vi "niRFUtil LCAPI Copy WFM (1 SGL).vi"(0 "Waveform In":T1 {"y" min=0 max=127 format="%.2f"; "dx" format="%^.2e"; "x0" format="%^.2e"}, 11 "error in (no error)":errorcluster, 12 "Data Copy Descriptor":u64, 13 "Ignore Data Copy Descriptor":bool) -> (4 "Waveform Out":T1 {"y" min=0 max=127 format="%.2f"; "dx" format="%^.2e"; "x0" format="%^.2e"}, 15 "error out":errorcluster)   [LabVIEW 2015, in "niRFUtil.lvlib"]
uses:
  niRFUtil.lvlib
  Includes/niRFUtil INC Real Waveform.ctl
  Includes/niRFUtil INC Real Array.ctl
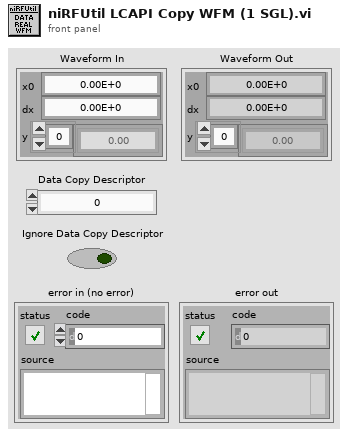
[diagram p1: front panel]
types:
  T1 = typedef "niRFUtil.lvlib/niRFUtil INC Real Waveform.ctl" = cluster{"x0":dbl, "dx":dbl, "y":T2}
  T2 = typedef "niRFUtil.lvlib/niRFUtil INC Real Array.ctl" = sgl[]
  T3 = cluster{"status":bool, "return type":i32, "errorString":string}
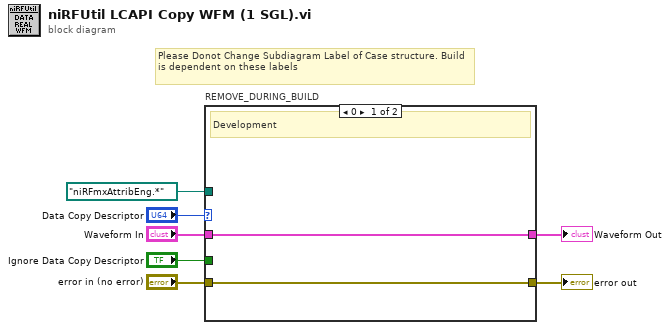
[diagram p0: block diagram]
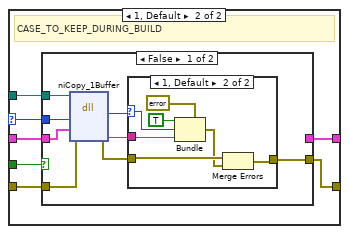
[diagram p2: hidden frame]
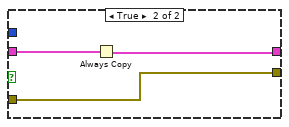
[diagram p4: hidden frame]
diagram:
  # "Please Donot Change Subdiagram Label of Case structure. Build is dependent on these labels"
  n1 = case "REMOVE_DURING_BUILD" shown="0" "Data Copy Descriptor" {
    selector: "Data Copy Descriptor" -> [_ w12]
    tunnel: "Waveform In" -> [w8 w16]
    tunnel: "error in (no error)" -> [w9 w15]
    tunnel: [w8 w14] -> w5
    tunnel: "Ignore Data Copy Descriptor" -> [_ w13]
    tunnel: [w9 w11] -> w2
    tunnel: path "niRFmxAttribEng.*" ("path in") -> [_ w10]
    frame 0 {
      # "Development"
    }
    frame 1, Default {
      # "CASE_TO_KEEP_DURING_BUILD"
      n2 = case shown="False" w13 {
        tunnel: w15 -> [w24 w35]
        tunnel: w16 -> [w23 w33]
        tunnel: w12 -> [w22 _]
        tunnel: [w18 w35] -> w11
        tunnel: [_ w34] -> w14
        tunnel: w10 -> [w17 _]
        frame False {
          n3 = dll-call lib="niRFmxAttribEng.*" fn="niCopy_1Buffer"(path in=w17, error in=w24, "dataCopyDescriptor"=w22, "source"=w23) -> (error out=w19:errorcluster, "return type"=w20:i32, "errorString"=w21:string)  [unwired: 4 in, 1 out]
          n4 = case shown="1, Default" w20 {
            selector: w20 -> [_ w30]
            tunnel: w21 -> [_ w31]
            tunnel: w19 -> [w25 w28]
            tunnel: [w25 w29] -> w18
            frame 0 {
            }
            frame 1, Default {
              n5 = Bundle(cluster=T3 {"status"=FALSE, "return type"=0, "errorString"=""}, "status"=TRUE, "return type"=w30, "errorString"=w31) -> (w27:T3)
              n6 = Merge Errors(w28, w27) -> (w29:errorcluster)
            }
          }
        }
        frame True {
          n7 = Always Copy(1:w33) -> (0:w34:T1)
        }
      }
    }
  }
  "error out" <- w2
  "Waveform Out" <- w5
